vi "Quick Scale 2D.vi"(0 "X":dbl[][](array[numeric]) format="%0.2f") -> (1 "Yij=Xij/Max|X|":dbl[][](array[numeric]) format="%0.2f", 2 "max|X|":dbl format="%0.2f", 3 "error":i32)   [LabVIEW 2014, in "NI_AALBase.lvlib"]
doc: "Determines the maximum absolute value of the input <B>X</B> and then scales <B>X</B> using this value."
uses:
  NI_AALBase.lvlib
  lvanlys.dll
panel:
  # "Yij=Xij/Max|X|"
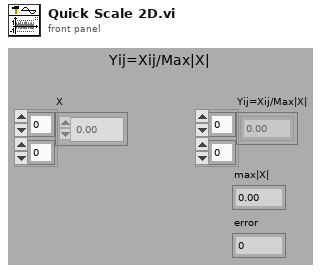
[diagram p1: front panel]
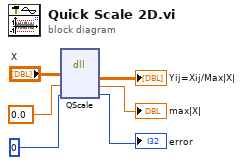
[diagram p0: block diagram]
diagram:
  n1 = dll-call lib="C:/Program Files (x86)/National Instruments/LabVIEW 2014/resource/lvanlys.*" fn="QScale"("X"="X", 0.0, 0) -> ("X"=→"Yij=Xij/Max|X|":dbl[][], →"max|X|":dbl, →"error":i32)  [unwired: 4 in, 2 out]
